vi "Мультиплексор класт.vi"(1 "МХ":bool, 2 "Cl 0":T2, 3 "Cl 1":T3) -> (0 "cl 2":T1)   [LabVIEW 2017]
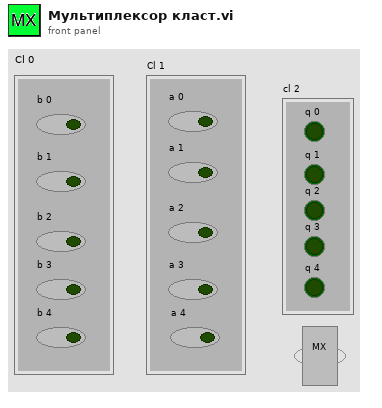
[diagram p1: front panel]
types:
  T1 = cluster{"q 0":bool, "q 1":bool, "q 2":bool, "q 3":bool, "q 4":bool}
  T2 = cluster{"b 0":bool, "b 1":bool, "b 2":bool, "b 3":bool, "b 4":bool}
  T3 = cluster{"a 0":bool, "a 1":bool, "a 2":bool, "a 3":bool, "a 4":bool}
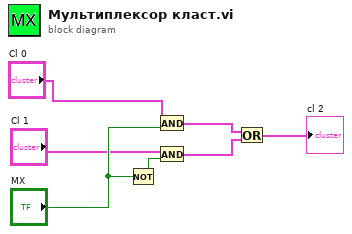
[diagram p0: block diagram]
diagram:
  n1 = Not(x="МХ") -> (.not. x?=w7:bool)
  n2 = And(x="Cl 0", y="МХ") -> (x .and. y?=w5:T2)
  n3 = And(x="Cl 1", y=w7) -> (x .and. y?=w4:T3)
  n4 = Or(x=w5, y=w4) -> (x .or. y?=→"cl 2":cluster{bool, bool, bool, bool, bool})
